vi "saturated MOSFET mobility.vi"() -> ()   [LabVIEW 2013]
uses:
  <vilib>/Analysis/baseanly.llb/Mean (DBL).vi
  <vilib>/Analysis/NI_AALBase.lvlib
panel:
  out "slope values used":dbl[](array[numeric])
  out "XY Graph":T1(graph)
  in  "Threshold Voltage (V)":dbl
  in  "Vg (V)           Id,sat (A)":dbl[][](array[numeric])
  out "Slope of  Id vs (Vg-Vth)^2":dbl format="%0.5f"
  out "Mobility (cm^2/Vs)":dbl
  in  "Length (m)":dbl=2.5e-05
  in  "Er for insulator (F/m)\n(3.9 for SiO2)":dbl=3.9
  in  "Thickness (m)":dbl=3e-07
  in  "Width (m)":dbl=0.002
  # "Saturation Current\nFET Mobility Calculator"
  # "Channel\nDimensions"
  # "Measurements"
  # "Gate Insulator"
  # "Results"
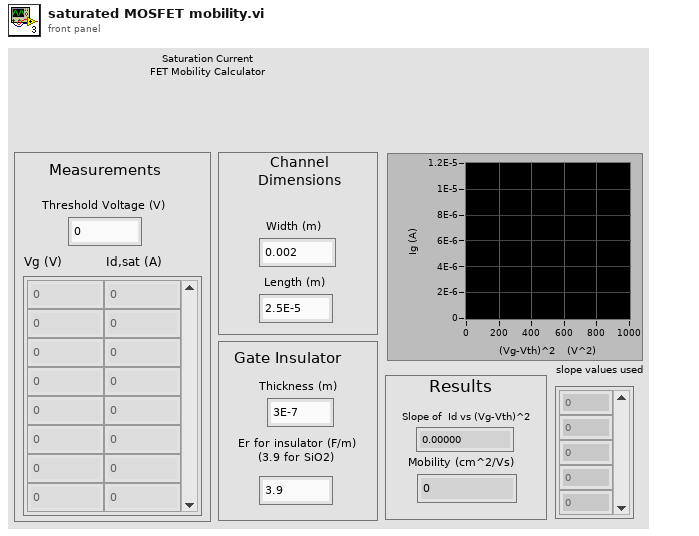
[diagram p1: front panel]
types:
  T1 = cluster{dbl[], "Vg (V)                 Id,sat (A)":dbl[]}
  T2 = cluster{dbl[], "Vg (V)           Id,sat (A)":dbl[]}
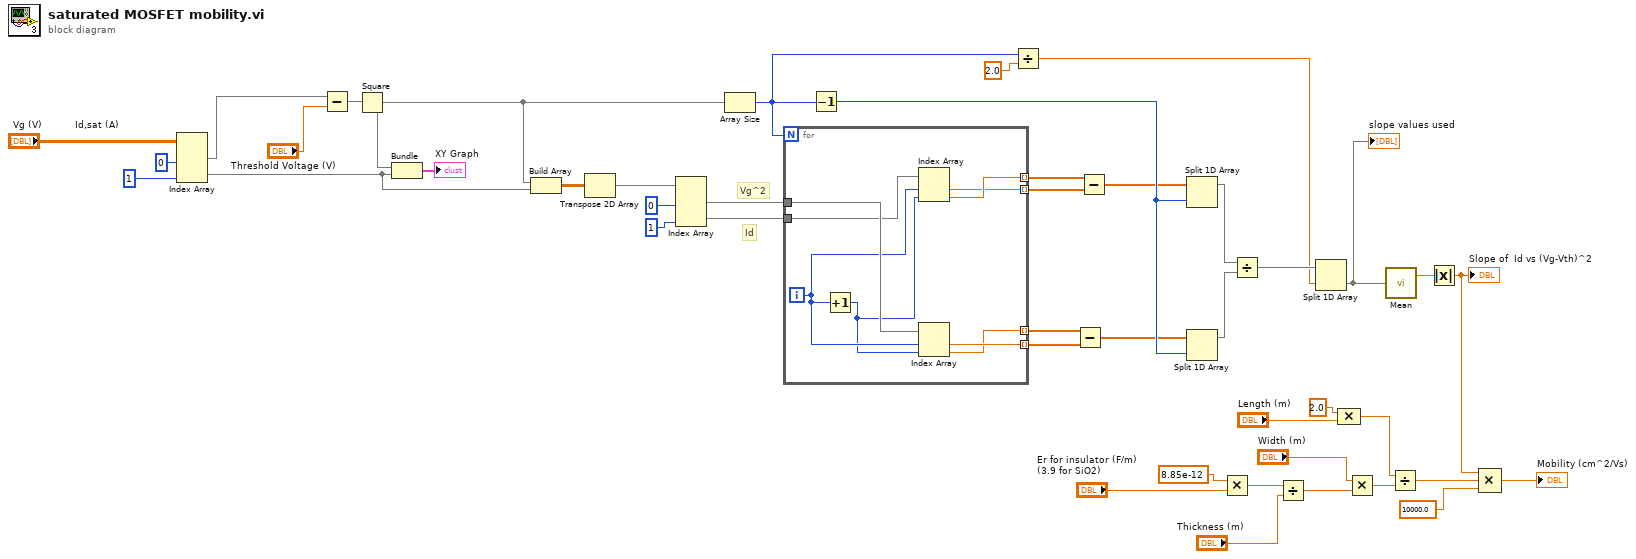
[diagram p0: block diagram]
diagram:
  # "Vg^2"
  # "Id"
  n1 = Index Array(array="Vg (V)           Id,sat (A)", index (col) #1=0 ("index (col)"), index (col) #2=1 ("index (col)")) -> (element #1=w15:dbl[], element #2=w13:dbl[])  [unwired: 2 in]
  n2 = Subtract(x=w15, y="Threshold Voltage (V)") -> (x-y=w14:dbl[])
  n3 = Square(x=w14) -> (x^2=w9:dbl[])
  n4 = Bundle(w9, "Vg (V)           Id,sat (A)"=w13) -> (→"XY Graph":T2)  [unwired: 1 in]
  n5 = Build Array(w9, w13) -> (w25:dbl[][])
  n6 = Transpose 2D Array(2D array=w25) -> (transposed array=w10:dbl[][])
  n7 = Index Array(array=w10, index (col) #1=0 ("index (row)"), index (col) #2=1 ("disabled index (col)")) -> (element #1=w8:dbl[], element #2=w28:dbl[])  [unwired: 2 in]
  n8 = Array Size(array=w9) -> (size(s)=w4:i32)
  n9 = for {
    N: w4 -> [_]
    tunnel: w8 -> [w52]
    tunnel: w28 -> [w51]
    tunnel: [w50] -> w33 mode=indexing
    tunnel: [w47] -> w34 mode=indexing
    tunnel: [w46] -> w32 mode=indexing
    tunnel: [w45] -> w31 mode=indexing
    i -> [w49]
    n10 = Increment(x=w49) -> (x+1=w48:i32)
    n11 = Index Array(array=w51, index #1=w49, index #2=w48) -> (element #1=w45:dbl, element #2=w46:dbl)
    n12 = Index Array(array=w52, index #1=w49, index #2=w48) -> (element #1=w50:dbl, element #2=w47:dbl)
  }
  n13 = Decrement(x=w4) -> (x-1=w30:i32)
  n14 = Divide(x=w4, y=2.0) -> (x/y=w1:dbl)
  n15 = Subtract(x=w34, y=w33) -> (x-y=w6:dbl[])
  n16 = Subtract(x=w32, y=w31) -> (x-y=w7:dbl[])
  n17 = Split 1D Array(array=w7, index=w30) -> (first subarray=w12:dbl[])  [unwired: 1 out]
  n18 = Split 1D Array(array=w6, index=w30) -> (first subarray=w11:dbl[])  [unwired: 1 out]
  n19 = Multiply(x=8.85e-12, y="Er for insulator (F/m)\n(3.9 for SiO2)") -> (x*y=w41:dbl)
  n20 = Divide(x=w12, y=w11) -> (x/y=w3:dbl[])
  n21 = Divide(x=w41, y="Thickness (m)") -> (x/y=w40:dbl)
  n22 = Split 1D Array(array=w3, index=w1) -> (second subarray=w2:dbl[])  [unwired: 1 out]
  "slope values used" <- w2
  n23 = Compound Arithmetic op=MULTIPLY(2.0 ("value"), "Length (m)") -> (w24:dbl)
  n24 = Multiply(x="Width (m)", y=w40) -> (x*y=w23:dbl)
  n25 = call-poly <vilib>:"Mean.vi"("X"=w2) -> ("mean"=w20:dbl)  [unwired: 1 out]
  n26 = Divide(x=w24, y=w23) -> (x/y=w18:dbl)
  n27 = Absolute Value(x=w20) -> (abs(x)=w19:dbl)
  "Slope of  Id vs (Vg-Vth)^2" <- w19
  n28 = Compound Arithmetic op=MULTIPLY(w19, w18, 10000.0 ("y")) -> (→"Mobility (cm^2/Vs)":dbl)
